vi "Flip2010.vi"() -> ()   [LabVIEW 2010]
uses:
  OpenCVWrapper.dll
panel:
  out "return":i32
  in  "Flip Mode":i32(ring) items=["Flip around x-axis"=0, "Flip around y-axis"=1, "Flip around both axis"=-1]
  out "Flipped Image":picture
  out "Original Picture":picture
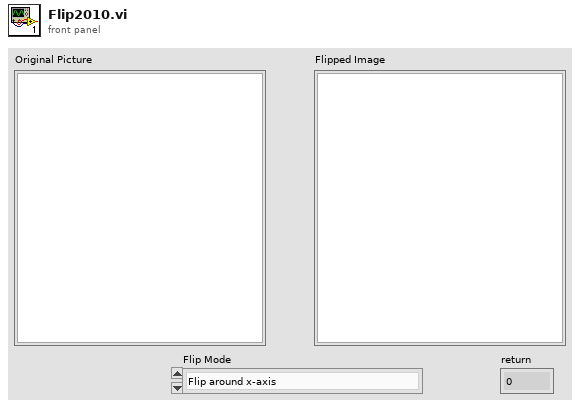
[diagram p1: front panel]
types:
  T1 = typedef "imagedata.ctl" = cluster{"image type":i32, "image depth":i32, "image":u8[], "mask":u8[], "colors":u32[], "Rectangle":cluster{"left":i16, "top":i16, "right":i16, "bottom":i16}}
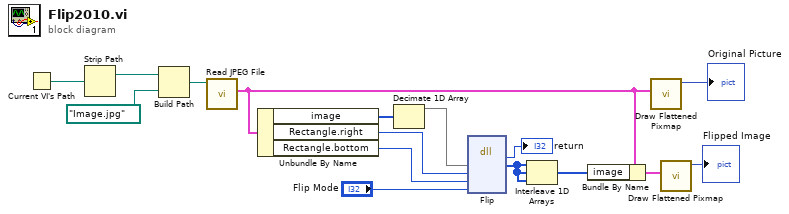
[diagram p0: block diagram]
diagram:
  n1 = Current VI's Path() -> (path=w6:path)
  n2 = Strip Path(path=w6) -> (stripped path=w5:path)  [unwired: 1 out]
  n3 = Build Path(base path=w5, name or relative path=path "Image.jpg") -> (appended path=w3:path)
  n4 = call <vilib>:"Read JPEG File.vi"("path to JPEG file"=w3) -> ("image data"=w2:T1)  [unwired: 8 in, 2 out]
  n5 = Unbundle By Name(w2) -> ("image"=w16:u8[], "Rectangle.right"=w13:i16, "Rectangle.bottom"=w12:i16)
  n6 = Decimate 1D Array(w16) -> (w14:u8[])  [unwired: 2 out]
  n7 = dll-call lib="C:/Users/108003658/OneDrive - Baker Hughes/Desktop/OpenCVDemo/OpenCVWrapper.dll" fn="Flip"("Image"=w14, "Width"=w13, "Height"=w12, "FlipMode"="Flip Mode") -> ("return type"=→"return":i32, "Image"=w8:u8[])  [unwired: 6 in, 2 out]
  n8 = Interleave 1D Arrays(w8, w8, w8) -> (w11:u8[])
  n9 = Bundle By Name(cluster=w2, "image"=w11) -> (w10:T1)
  n10 = call <vilib>:"Draw Flattened Pixmap.vi"("image data"=w2) -> ("new picture"=→"Original Picture":picture)  [unwired: 8 in]
  n11 = call <vilib>:"Draw Flattened Pixmap.vi"("image data"=w10) -> ("new picture"=→"Flipped Image":picture)  [unwired: 8 in]
